vi "line scan enable disable.vi"(11 "Page Enabled State":T1(ring)) -> ()   [LabVIEW 2012]
uses:
  GFG/GFGfpRefGet.vi
  GFG/GFG library.lvlib
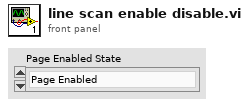
[diagram p1: front panel]
types:
  T1 = enum32{"Page Enabled", "Page Disabled", "Page Disabled & Grayed"}
  T2 = cluster{"WaveformChartRef":refnum<vi>, "DigitalRef":refnum<vi>, "ArrayRef":refnum<vi>, "TabControlRef":refnum<vi>, "EnumRef":refnum<vi>, "RingRef":refnum<vi>, "BooleanRef":refnum<vi>, "KnobRef":refnum<vi>, "SlideRef":refnum<vi>, "PathRef":refnum<vi>, "StringRef":refnum<vi>, "ComboBox":refnum<vi>, "WaveformGraphRef":refnum<vi>}
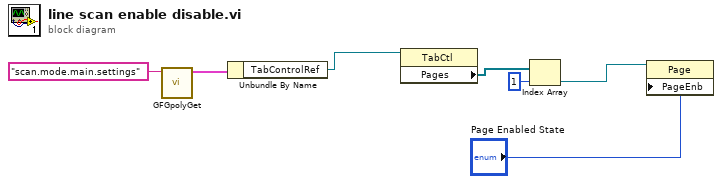
[diagram p0: block diagram]
diagram:
  n1 = call-poly "GFGpolyGet.vi"("Variable Name in"="scan.mode.main.settings") -> ("output cluster"=w7:T2)  [unwired: 9 in, 1 out]
  n2 = Unbundle By Name(w7) -> ("TabControlRef"=w5:refnum<vi>)
  n3 = property class="TabCtl"(reference=w5) -> ("Pages"=w4:refnum<vi>[])  [unwired: 1 in, 2 out]
  n4 = Index Array(array=w4, index=1) -> (element=w2:refnum<vi>)
  n5 = property class="Page"(reference=w2, "PageEnb"="Page Enabled State") -> ()  [unwired: 1 in, 2 out]
